vi "ObtainPrefixQueue.vi"(5 "Max Queue Size (-1, Unlimited)":i32=-1, 7 "Create If Not Found? (T)":bool=TRUE, 8 "error in (no error)":errorcluster, 11 "Queue Name":string) -> (0 "error out":errorcluster, 1 "Created New?":bool, 3 "PrefixQueue out":refnum<class "PrefixQueue.lvclass">)   [LabVIEW 2017, in "LapDog.Messaging.v3.PrefixQueue.lvlib" / "PrefixQueue.lvclass"]
doc: "Returns a fully configured PrefixQueue object.\n\nA PrefixQueue is a specific kind of MessageQueue that allows a standard prefix to be prepended to the names of all messages enqueued on that branch of the queue."
uses:
  PrefixQueue.lvclass
  PrefixQueue.lvclass/PrefixQueue.ctl
panel:
  in  "Message Name Prefix":string
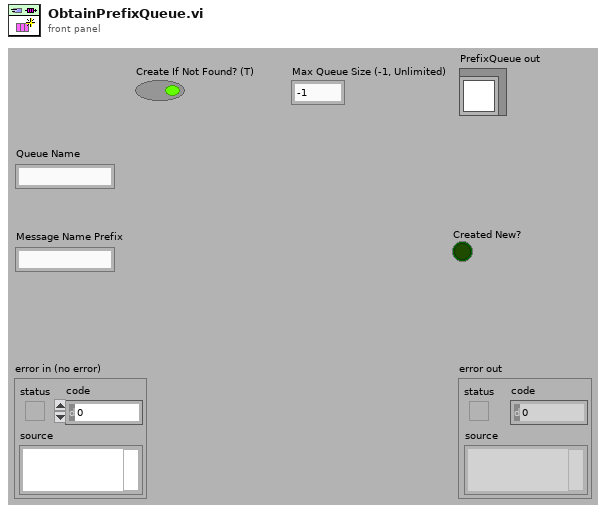
[diagram p1: front panel]
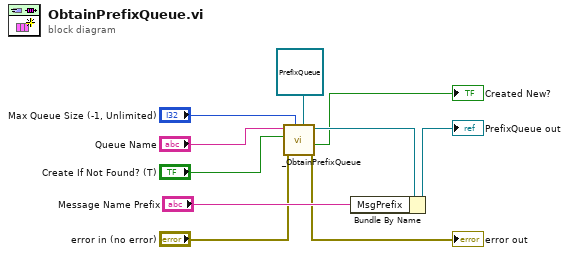
[diagram p0: block diagram]
diagram:
  n1 = call "_ObtainPrefixQueue.vi"("PrefixQueue Type"=refnum<class "PrefixQueue.lvclass"> refnum ("PrefixQueue"), "Max Queue Size (-1, Unlimited)"="Max Queue Size (-1, Unlimited)", "error in (no error)"="error in (no error)", "Create If Not Found? (T)"="Create If Not Found? (T)", "Queue Name"="Queue Name") -> ("error out"=→"error out":errorcluster, "Created New?"=→"Created New?":bool, "PrefixQueue out"=w7:refnum<class "PrefixQueue.lvclass">)  [unwired: 4 in]
  n2 = Bundle By Name(cluster=w7, "MsgPrefix"="Message Name Prefix") -> (→"PrefixQueue out":refnum<class "PrefixQueue.lvclass">)
